vi "Connect Core.vi"(6 "Access (R/W allowed)":T1, 8 "error in (no error)":errorcluster, 11 "DIMConnection in":refnum<class "DIMConnection.lvclass">) -> (0 "error out":errorcluster, 3 "DIMConnection out":refnum<class "DIMConnection.lvclass">)   [LabVIEW 2014, in "CS++DIM.lvlib" / "DIMConnection.lvclass"]
doc: "Opene reference to a process variable."
uses:
  DIMConnection.lvclass
  DimLVEvent/LVDimInterface/LVDimInterface.lvlib
  CSPP_Core/Classes/CS++ProcessVariables/PVConnection/PVConnection.lvclass
  CSPP_Core/Classes/CS++ProcessVariables/ProcessVariable/PV.lvclass
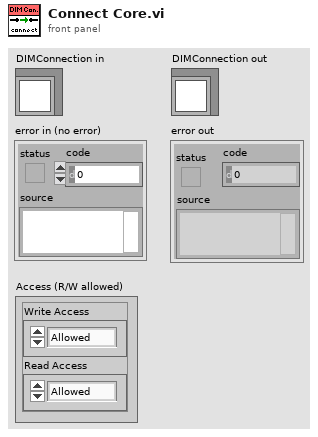
[diagram p1: front panel]
types:
  T1 = cluster{"Write Access":enum8{"Allowed", "Required", "None"}, "Read Access":enum8{"Allowed", "Required", "None"}}
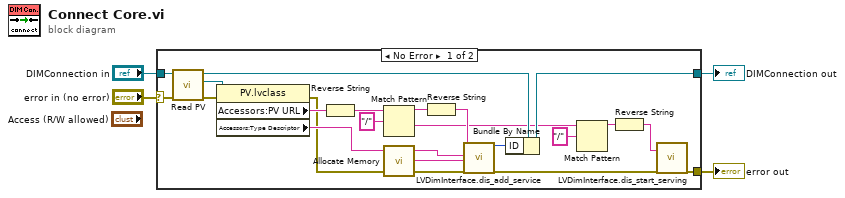
[diagram p0: block diagram]
diagram:
  n1 = case shown="No Error" "error in (no error)" {
    selector: "error in (no error)" -> [w20 w29]
    tunnel: "DIMConnection in" -> [w27 w28]
    tunnel: [w15 w29] -> w3
    tunnel: [w22 w28] -> w2
    frame No Error {
      n2 = call "Read PV.vi"("error in (no error)"=w20, "PVConnection in"=w27) -> ("error out"=w25:errorcluster, "PV"=w26:refnum<class "PV.lvclass">, "PVConnection out"=w24:refnum<class "DIMConnection.lvclass">)  [unwired: 7 in]
      n3 = property class="PV.lvclass"(reference=w26, error in=w25) -> (error out=w6:errorcluster, "Accessors:PV URL"=w13:string, "Accessors:Type Descriptor"=w19:string)  [unwired: 1 out]
      n4 = Reverse String(1:w13) -> (0:w14:string)
      n5 = Match Pattern(string=w14, regular expression="/" ("search string/char (-)")) -> (before substring=w12:string, after substring=w10:string)  [unwired: 1 in, 2 out]
      n6 = call "Allocate Memory.vi"("Error In"=w6, "Type Descriptor"=w19) -> ("Error Out"=w5:errorcluster, "Data"=w17:string, "dup Type Descriptor"=w18:string)  [unwired: 1 in]
      n7 = Reverse String(1:w12) -> (0:w11:string)
      n8 = call "LVDimInterface.dis_add_service.vi"("serviceName"=w11, "typeDescriptor"=w18, "data"=w17, "error in (no error)"=w5) -> ("my_serviceID"=w23:i32, "error out"=w16:errorcluster)  [unwired: 14 in]
      n9 = Bundle By Name(cluster=w24, "ID"=w23) -> (w22:refnum<class "DIMConnection.lvclass">)
      n10 = Match Pattern(string=w10, regular expression="/") -> (before substring=w9:string)  [unwired: 1 in, 3 out]
      n11 = Reverse String(1:w9) -> (0:w8:string)
      n12 = call "LVDimInterface.dis_start_serving.vi"("serverName"=w8, "error in (no error)"=w16) -> ("error out"=w15:errorcluster)  [unwired: 16 in, 1 out]
    }
    frame Error {
    }
  }
  "error out" <- w3
  "DIMConnection out" <- w2
